vi "Run_Python_Command.vi"(8 "error in":errorcluster, 10 "name or relative path":path, 11 "Functions":T1=enum."HMS_IPConfig_Conflict_IP") -> (0 "error out":errorcluster, 2 "Standard Output":string, 3 "Output":bool)   [LabVIEW 2025]
uses:
  Control/Python Function.ctl
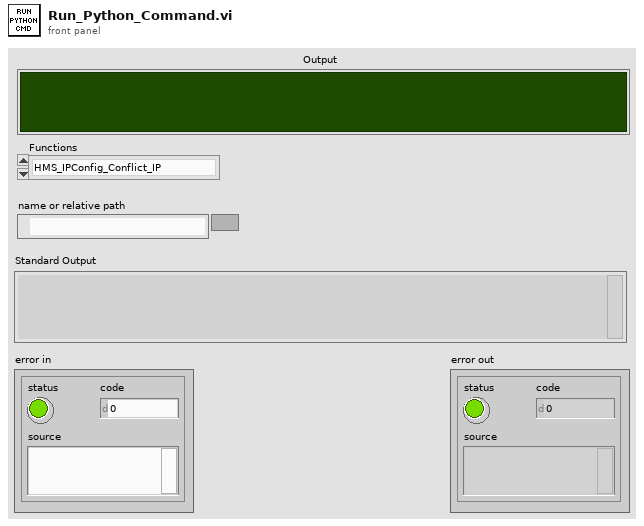
[diagram p1: front panel]
types:
  T1 = typedef "Python Function.ctl" = enum16{"HMS_IPConfig", "HMS_IPConfig_Verify_DHCP_Enabled", "HMS_IPConfig_Conflict_IP", "Verify Input Voltage", "Verify Battery Voltage", "Verify Output Voltage", "Verify Output Current"}
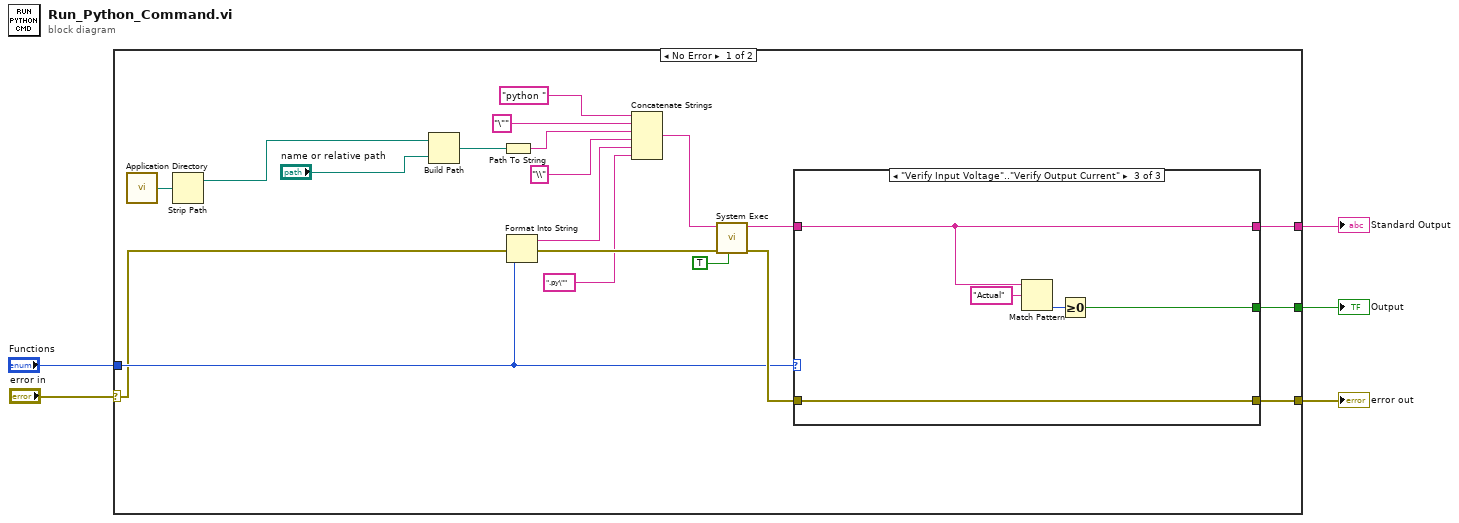
[diagram p0: block diagram]
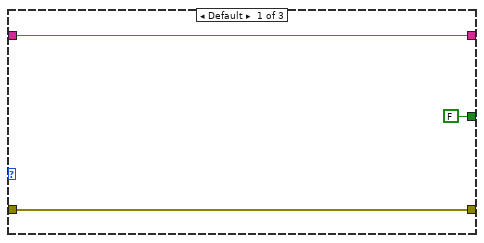
[diagram p2: hidden frame]
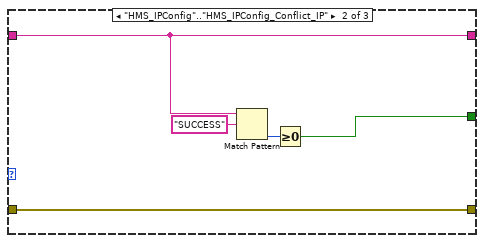
[diagram p3: hidden frame]
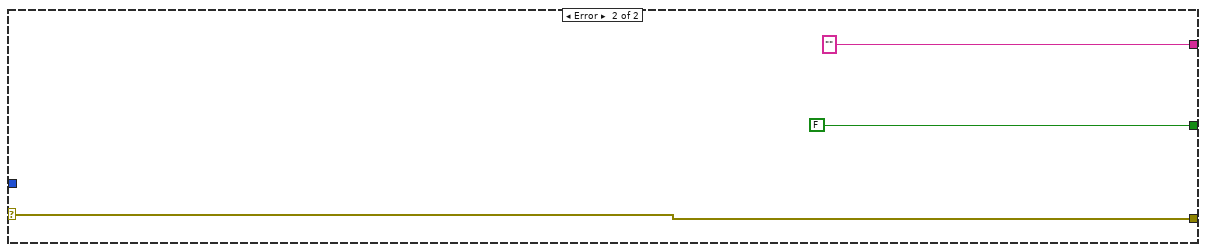
[diagram p4: hidden frame]
diagram:
  n1 = case shown="No Error" "error in" {
    selector: "error in" -> [w7 w41]
    tunnel: [w19 w41] -> w4
    tunnel: "Functions" -> [w18 _]
    tunnel: [w16 "" ("standard output")] -> w3
    tunnel: [w17 FALSE] -> w2
    frame No Error {
      n2 = call <vilib>:"Application Directory.vi"() -> ("Application Directory"=w25:path)
      n3 = Strip Path(path=w25) -> (stripped path=w14:path)  [unwired: 1 out]
      n4 = Build Path(base path=w14, name or relative path="name or relative path") -> (appended path=w23:path)
      n5 = Path To String(path=w23) -> (string=w24:string)
      n6 = Format Into String(error in=w7, w18) -> (resulting string=w12:string, error out=w21:errorcluster)  [unwired: 2 in]
      n7 = Concatenate Strings("python " ("string"), "\"" ("string"), w24, "\\" ("string"), w12, ".py\"" ("string")) -> (w8:string)
      n8 = call <vilib>:"System Exec.vi"("run minimized? (F)"=TRUE, "error in (no error)"=w21, "command line"=w8) -> ("error out"=w20:errorcluster, "standard output"=w15:string)  [unwired: 5 in, 2 out]
      n9 = case shown="\"Verify Input Voltage\"..\"Verify Output Current\"" w18 {
        tunnel: [FALSE w30 w35] -> w17
        tunnel: w20 -> [w28 w31 w36]
        tunnel: [w28 w31 w36] -> w19
        tunnel: [w27 w29 w34] -> w16
        tunnel: w15 -> [w27 w29 w34]
        frame Default {
        }
        frame "HMS_IPConfig".."HMS_IPConfig_Conflict_IP" {
          n10 = Match Pattern(string=w29, regular expression="SUCCESS") -> (offset past match=w32:i32)  [unwired: 1 in, 3 out]
          n11 = Greater Or Equal To 0?(x=w32) -> (x >= 0?=w30:bool)
        }
        frame "Verify Input Voltage".."Verify Output Current" {
          n12 = Match Pattern(string=w34, regular expression="Actual") -> (offset past match=w37:i32)  [unwired: 1 in, 3 out]
          n13 = Greater Or Equal To 0?(x=w37) -> (x >= 0?=w35:bool)
        }
      }
    }
    frame Error {
    }
  }
  "error out" <- w4
  "Standard Output" <- w3
  "Output" <- w2
